vi "Cholesky Factorization Rank-1 Update_Update (CDB).vi"(10 "X":cdb[](array[numeric]), 11 "R":T1) -> (3 "Updated R":T1)   [LabVIEW 2020, in "NI_AAL_LinAlg.lvlib"]
uses:
  <vilib>/Analysis/NI_AAL_LinAlg.lvlib
  <vilib>/Analysis/Matrix/Datatypes/ComplexMatrix.ctl
  <vilib>/Analysis/Matrix/NI_Matrix.lvlib
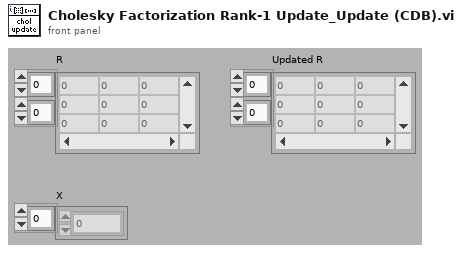
[diagram p1: front panel]
types:
  T1 = typedef "NI_Matrix.lvlib/ComplexMatrix.ctl" = cdb[][]
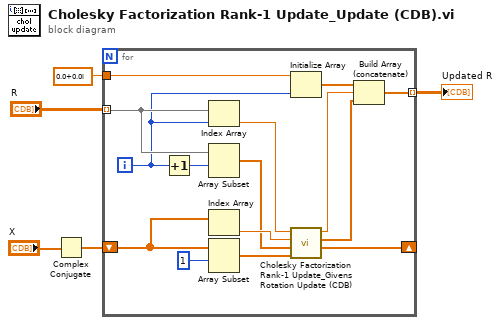
[diagram p0: block diagram]
diagram:
  n1 = Complex Conjugate(1:"X") -> (0:w4:cdb[])
  n2 = for {
    shift-right: [w6] -> _
    shift-left: w4 -> [w19]
    tunnel: "R" -> [w18] mode=indexing
    tunnel: [w15] -> w1 mode=indexing
    tunnel: cdb 0.0+0.0i -> [w8]
    i -> [w14]
    n3 = Increment(x=w14) -> (x+1=w17:i32)
    n4 = Index Array(array=w18, index=w14) -> (element=w13:cdb)
    n5 = Array Subset(array=w18, index=w17) -> (w10:cdb[])  [unwired: 1 in]
    n6 = Index Array(array=w19) -> (element=w12:cdb)  [unwired: 1 in]
    n7 = Array Subset(array=w19, index=1) -> (w11:cdb[])  [unwired: 1 in]
    n8 = Initialize Array(w8, w14) -> (w20:cdb[])
    n9 = call <vilib>:"Cholesky Factorization Rank-1 Update_Givens Rotation Update (CDB).vi"("Y In"=w11, "X In"=w10, "b"=w12, "a"=w13) -> ("Y Out"=w6:cdb[], "X Out"=w7:cdb[], "v"=w9:cdb)  [unwired: 5 in]
    n10 = Build Array (concatenate)(w20, w9, w7) -> (w15:cdb[])
  }
  "Updated R" <- w1
